vi "add scan PZT V(SubVI).vi"(10 "字符串":string) -> (1 "ok or cancel":bool, 2 "连接的字符串":string)   [LabVIEW 2019, in "nematic.lvlib"]
uses:
  nematic.lvlib
panel:
  in  "电压2":dbl=148.0
  in  "steps":dbl
  in  "电压1":dbl
  in  "cancel":bool
  in  "ok":bool
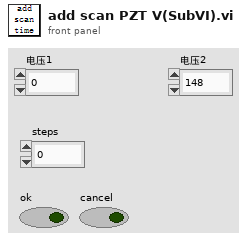
[diagram p1: front panel]
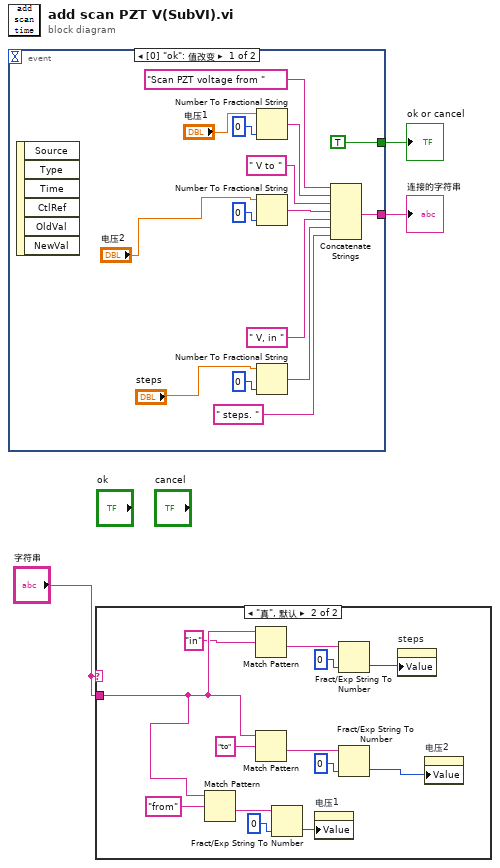
[diagram p0: block diagram]
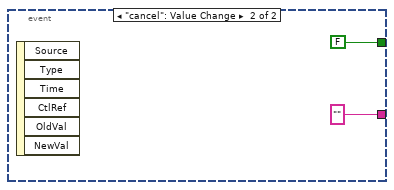
[diagram p3: hidden frame]
diagram:
  n1 = event shown="[0] \"ok\": 值改变" {
    selector: _ -> [_ _]
    dyn-events: _ -> [_ _]
    timeout: _ -> [_ _]
    tunnel: [TRUE FALSE] -> w2
    tunnel: [w11 "" ("分隔符")] -> w3
    event "ok": Value Change {
      n2 = event-data() -> ()  [unwired: 1 in, 6 out]
      n3 = Number To Fractional String(number="电压1", precision (6)=i16 0 ("精度(6)")) -> (F-format string=w16:string)  [unwired: 2 in]
      n4 = Number To Fractional String(number="电压2", precision (6)=i16 0 ("精度(6)")) -> (F-format string=w12:string)  [unwired: 2 in]
      n5 = Number To Fractional String(number="steps", precision (6)=i16 0 ("精度(6)")) -> (F-format string=w7:string)  [unwired: 2 in]
      n6 = Concatenate Strings("Scan PZT voltage from " ("字符串"), w16, " V to " ("字符串"), w12, " V, in " ("字符串"), w7, " steps. " ("string")) -> (w11:string)
    }
    event "cancel": Value Change {
      n7 = event-data() -> ()  [unwired: 1 in, 6 out]
    }
  }
  "ok or cancel" <- w2
  "连接的字符串" <- w3
  n8 = case shown="\"真\", 默认" "字符串" {
    tunnel: "字符串" -> [_ w29]
    frame "" {
    }
    frame "真", Default {
      n9 = Match Pattern(string=w29, regular expression="from" ("正则表达式")) -> (after substring=w31:string)  [unwired: 1 in, 3 out]
      n10 = Match Pattern(string=w29, regular expression="in" ("正则表达式")) -> (after substring=w24:string)  [unwired: 1 in, 3 out]
      n11 = Match Pattern(string=w29, regular expression="to" ("正则表达式")) -> (after substring=w25:string)  [unwired: 1 in, 3 out]
      n12 = Fract/Exp String To Number(string=w31, default (0 dbl)=0) -> (number=w23:i32)  [unwired: 2 in, 1 out]
      n13 = property on="电压1" class="DigNum (严格)"("Value"=w23) -> ()  [unwired: 2 in, 2 out]
      n14 = Fract/Exp String To Number(string=w24, default (0 dbl)=0) -> (number=w22:i32)  [unwired: 2 in, 1 out]
      n15 = Fract/Exp String To Number(string=w25, default (0 dbl)=0) -> (number=w21:i32)  [unwired: 2 in, 1 out]
      n16 = property on="steps" class="DigNum (严格)"("Value"=w22) -> ()  [unwired: 2 in, 2 out]
      n17 = property on="电压2" class="DigNum (严格)"("Value"=w21) -> ()  [unwired: 2 in, 2 out]
    }
  }
